vi "WPI_CAN_PDPReceive.vi"(11 "Power Distribution Panel (0)":u8) -> (3 "Power Distribution Panel Out":u8)   [LabVIEW 2017]
uses:
  <vilib>/Rock Robotics/WPI/CAN/PDP/WPI_CAN_PDPMessageIDs.ctl
  <vilib>/Rock Robotics/WPI/CAN/PDP/WPI_CAN_PDPGetAll.ctl
  <vilib>/Rock Robotics/WPI/CAN/PDP/WPI_CAN_PDPGlobalOps.ctl
panel:
  out "Tmeas (ms)":u8
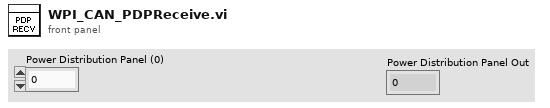
[diagram p1: front panel]
types:
  T1 = typedef "WPI_CAN_PDPMessageIDs.ctl" = u32
  T2 = typedef "WPI_CAN_PDPGetAll.ctl" = cluster{"Channel Currents":dbl[], "Battery Voltage":dbl, "Temperature (degrees C)":dbl, "Internal Battery R (Ohms)":dbl, "Energy (J)":dbl, "Power (W)":dbl, "Total Current (A)":dbl, "CAN Error":errorcluster, "Current Faults":bool[], "Battery Voltage Fault":bool, "Temperature Fault":bool, "Hardware Fault":bool}
  T3 = typedef "WPI_CAN_PDPGlobalOps.ctl" = enum16{"Write After Receive 0-5", "Write After Receive 6-11", "Write After Receive 12-15", "Write After Receive Energy", "Get All", "Get Commands", "Write Clear Sticky Faults Command", "Write Reset Energy Command", "Write Tare Currents Command", "Write Error", "Write After Receive Faults"}
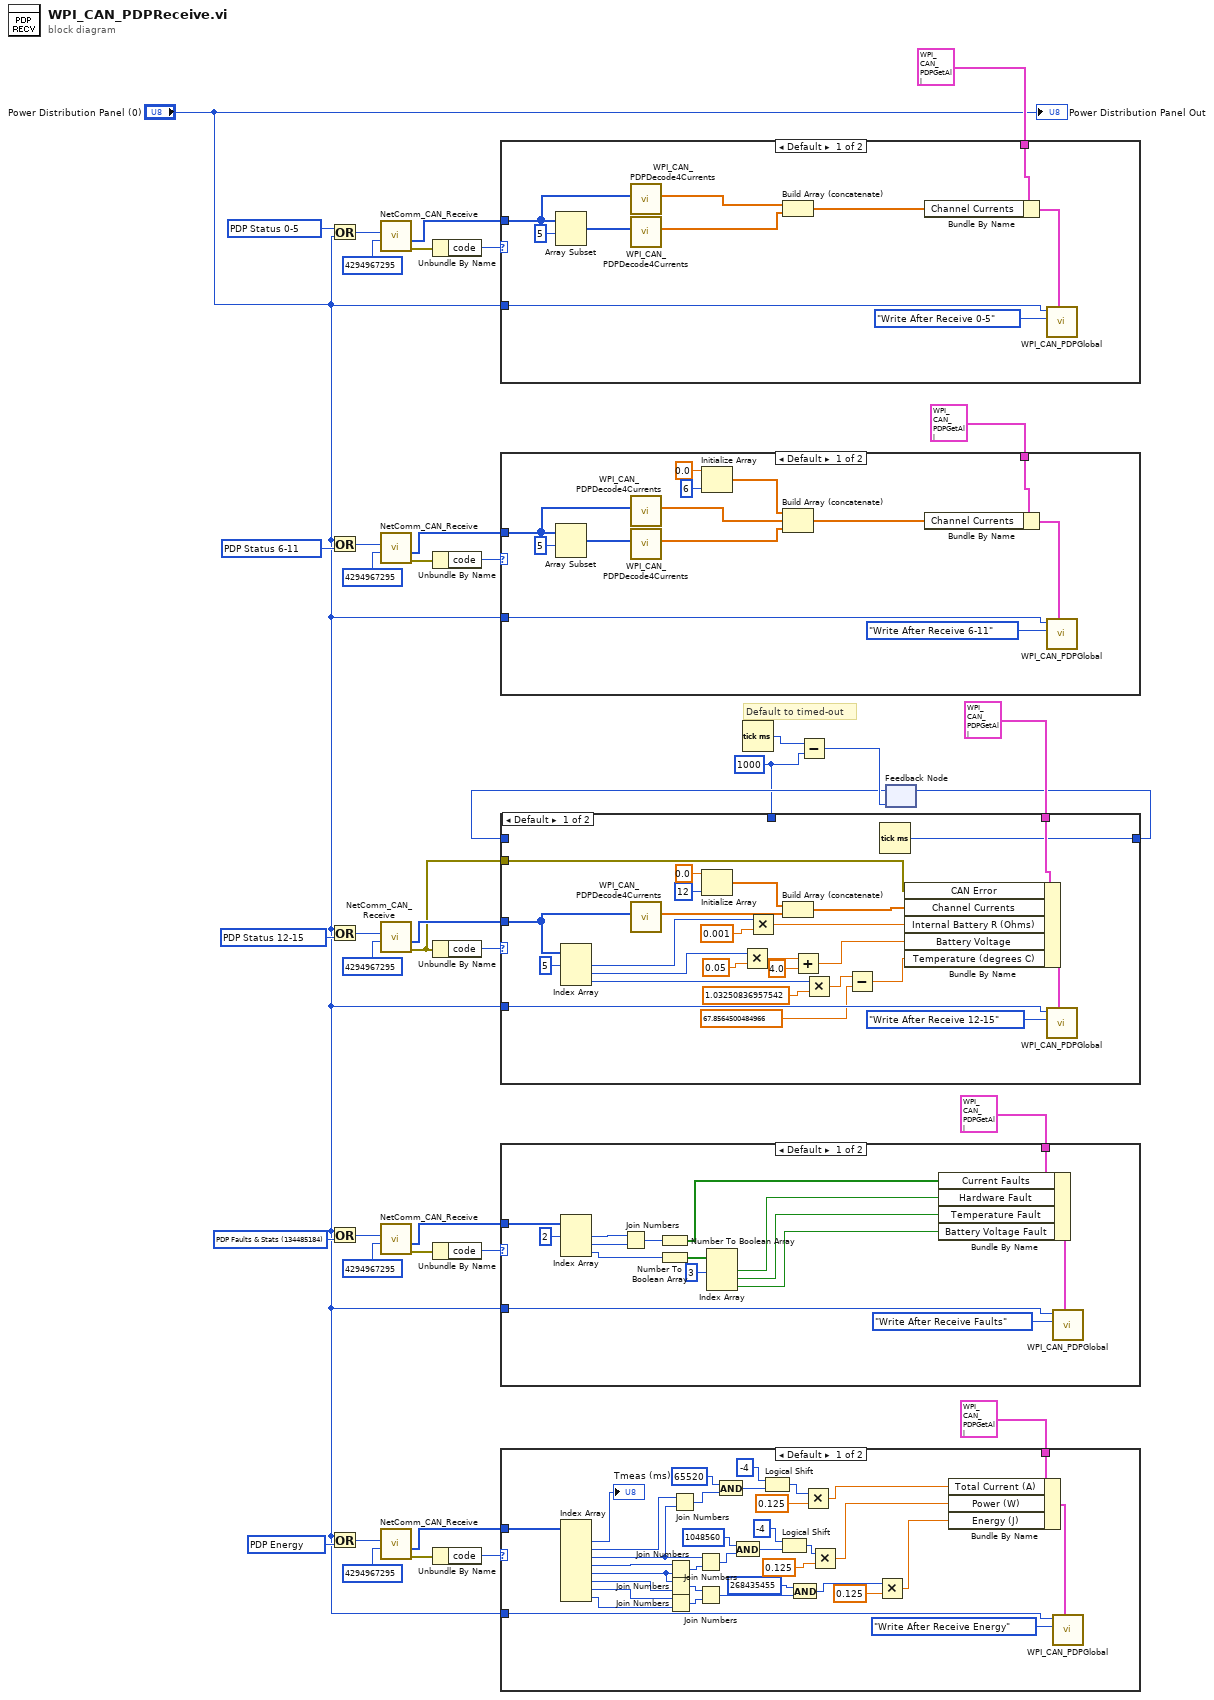
[diagram p0: block diagram]
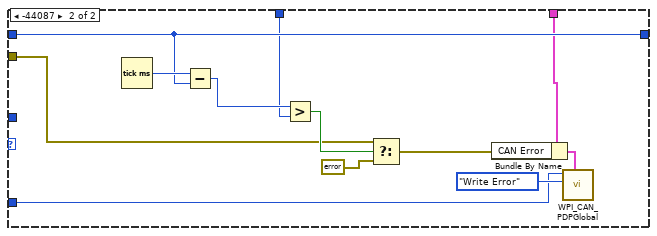
[diagram p4: hidden frame]
diagram:
  w2 = T1 134485184 items=["PDP Status 0-5"=134484992, "PDP Status 6-11"=134485056, "PDP Status 12-15"=134485120, "PDP Faults & Stats"=134485184, "PDP Energy"=134485824, "PDP Commands"=134487040, "PDP Update Event"=134487168, "PDP Update Robot State"=134487104] ("PDP Message IDs")
  w9 = u32 1000 ("y")
  w20 = T1 134485824 items=["PDP Status 0-5"=134484992, "PDP Status 6-11"=134485056, "PDP Status 12-15"=134485120, "PDP Faults & Stats"=134485184, "PDP Energy"=134485824, "PDP Commands"=134487040, "PDP Update Event"=134487168, "PDP Update Robot State"=134487104] ("PDP Message IDs")
  w21 = T1 134485120 items=["PDP Status 0-5"=134484992, "PDP Status 6-11"=134485056, "PDP Status 12-15"=134485120, "PDP Faults & Stats"=134485184, "PDP Energy"=134485824, "PDP Commands"=134487040, "PDP Update Event"=134487168, "PDP Update Robot State"=134487104] ("PDP Message IDs")
  w22 = T1 134485056 items=["PDP Status 0-5"=134484992, "PDP Status 6-11"=134485056, "PDP Status 12-15"=134485120, "PDP Faults & Stats"=134485184, "PDP Energy"=134485824, "PDP Commands"=134487040, "PDP Update Event"=134487168, "PDP Update Robot State"=134487104] ("PDP Message IDs")
  w23 = T1 134484992 items=["PDP Status 0-5"=134484992, "PDP Status 6-11"=134485056, "PDP Status 12-15"=134485120, "PDP Faults & Stats"=134485184, "PDP Energy"=134485824, "PDP Commands"=134487040, "PDP Update Event"=134487168, "PDP Update Robot State"=134487104] ("PDP Message IDs")
  # "Default to timed-out"
  n1 = Or(x=w23, y="Power Distribution Panel (0)") -> (x .or. y?=w41:T1)
  n2 = Or(x="Power Distribution Panel (0)", y=w22) -> (x .or. y?=w25:T1)
  n3 = Or(x="Power Distribution Panel (0)", y=w21) -> (x .or. y?=w24:T1)
  n4 = Or(x="Power Distribution Panel (0)", y=w2) -> (x .or. y?=w3:T1)
  n5 = Or(x="Power Distribution Panel (0)", y=w20) -> (x .or. y?=w19:T1)
  n6 = call <vilib>:"NetComm_CAN_Receive.vi"("Message ID Mask"=u32 4294967295, "Message ID"=w41) -> ("error out"=w39:errorcluster, "Data"=w33:u8[])  [unwired: 6 in, 2 out]
  n7 = call <vilib>:"NetComm_CAN_Receive.vi"("Message ID Mask"=u32 4294967295, "Message ID"=w25) -> ("error out"=w37:errorcluster, "Data"=w35:u8[])  [unwired: 6 in, 2 out]
  n8 = call <vilib>:"NetComm_CAN_Receive.vi"("Message ID Mask"=u32 4294967295, "Message ID"=w24) -> ("error out"=w26:errorcluster, "Data"=w31:u8[])  [unwired: 6 in, 2 out]
  n9 = call <vilib>:"NetComm_CAN_Receive.vi"("Message ID Mask"=u32 4294967295, "Message ID"=w3) -> ("error out"=w4:errorcluster, "Data"=w8:u8[])  [unwired: 6 in, 2 out]
  n10 = call <vilib>:"NetComm_CAN_Receive.vi"("Message ID Mask"=u32 4294967295, "Message ID"=w19) -> ("error out"=w18:errorcluster, "Data"=w14:u8[])  [unwired: 6 in, 2 out]
  n11 = Unbundle By Name(w39) -> ("code"=w34:i32)
  n12 = Unbundle By Name(w37) -> ("code"=w36:i32)
  n13 = Unbundle By Name(w26) -> ("code"=w30:i32)
  n14 = Unbundle By Name(w4) -> ("code"=w7:i32)
  n15 = Unbundle By Name(w18) -> ("code"=w15:i32)
  n16 = case shown="Default" w34 {
    tunnel: "Power Distribution Panel (0)" -> [w50 _]
    tunnel: w33 -> [w43 _]
    tunnel: T2 {"Channel Currents"=[], "Battery Voltage"=0.0, "Temperature (degrees C)"=0.0, "Internal Battery R (Ohms)"=0.0, "Energy (J)"=0.0, "Power (W)"=0.0, "Total Current (A)"=0.0, "CAN Error"={"status"=FALSE, "code"=0, "source"=""}, "Current Faults"=[], "Battery Voltage Fault"=FALSE, "Temperature Fault"=FALSE, "Hardware Fault"=FALSE} ("Write After Receive") -> [w42 _]
    frame Default {
      n17 = Array Subset(array=w43, index=5) -> (w47:u8[])  [unwired: 1 in]
      n18 = call <vilib>:"WPI_CAN_PDPDecode4Currents.vi"("5-Byte Array"=w43) -> ("4-Current Array"=w45:dbl[])  [unwired: 10 in]
      n19 = call <vilib>:"WPI_CAN_PDPDecode4Currents.vi"("5-Byte Array"=w47) -> ("4-Current Array"=w46:dbl[])  [unwired: 10 in]
      n20 = Build Array (concatenate)(w45, w46) -> (w44:dbl[])
      n21 = Bundle By Name(cluster=w42, "Channel Currents"=w44) -> (w49:T2)
      n22 = call <vilib>:"WPI_CAN_PDPGlobal.vi"("Write After Receive"=w49, "Operation"=WPI_CAN_PDPGlobalOps."Write After Receive 0-5", "Power Distribution Panel (0)"=w50) -> ()  [unwired: 6 in, 3 out]
    }
    frame -44087 {
    }
  }
  n23 = case shown="Default" w36 {
    tunnel: w35 -> [w59 _]
    tunnel: "Power Distribution Panel (0)" -> [w63 _]
    tunnel: T2 {"Channel Currents"=[], "Battery Voltage"=0.0, "Temperature (degrees C)"=0.0, "Internal Battery R (Ohms)"=0.0, "Energy (J)"=0.0, "Power (W)"=0.0, "Total Current (A)"=0.0, "CAN Error"={"status"=FALSE, "code"=0, "source"=""}, "Current Faults"=[], "Battery Voltage Fault"=FALSE, "Temperature Fault"=FALSE, "Hardware Fault"=FALSE} ("Write After Receive") -> [w62 _]
    frame Default {
      n24 = Array Subset(array=w59, index=5) -> (w58:u8[])  [unwired: 1 in]
      n25 = call <vilib>:"WPI_CAN_PDPDecode4Currents.vi"("5-Byte Array"=w59) -> ("4-Current Array"=w54:dbl[])  [unwired: 10 in]
      n26 = call <vilib>:"WPI_CAN_PDPDecode4Currents.vi"("5-Byte Array"=w58) -> ("4-Current Array"=w56:dbl[])  [unwired: 10 in]
      n27 = Initialize Array(0.0 ("element"), 6 ("dimension size")) -> (w55:dbl[])
      n28 = Build Array (concatenate)(w55, w54, w56) -> (w52:dbl[])
      n29 = Bundle By Name(cluster=w62, "Channel Currents"=w52) -> (w61:T2)
      n30 = call <vilib>:"WPI_CAN_PDPGlobal.vi"("Write After Receive"=w61, "Operation"=WPI_CAN_PDPGlobalOps."Write After Receive 6-11", "Power Distribution Panel (0)"=w63) -> ()  [unwired: 6 in, 3 out]
    }
    frame -44087 {
    }
  }
  n31 = case shown="Default" w7 {
    tunnel: w8 -> [w76 _]
    tunnel: "Power Distribution Panel (0)" -> [w79 _]
    tunnel: T2 {"Channel Currents"=[], "Battery Voltage"=0.0, "Temperature (degrees C)"=0.0, "Internal Battery R (Ohms)"=0.0, "Energy (J)"=0.0, "Power (W)"=0.0, "Total Current (A)"=0.0, "CAN Error"={"status"=FALSE, "code"=0, "source"=""}, "Current Faults"=[], "Battery Voltage Fault"=FALSE, "Temperature Fault"=FALSE, "Hardware Fault"=FALSE} ("Write After Receive") -> [w78 _]
    frame Default {
      n32 = Index Array(array=w76, index #1=2 ("index")) -> (element #1=w75:u8, element #2=w74:u8, element #3=w70:u8)  [unwired: 2 in]
      n33 = Join Numbers(hi=w75, lo=w74) -> ((hi.lo)=w73:u16)
      n34 = Number To Boolean Array(number=w73) -> (Boolean array=w72:bool[])
      n35 = Number To Boolean Array(number=w70) -> (Boolean array=w69:bool[])
      n36 = Index Array(array=w69, index #1=3 ("index")) -> (element #1=w67:bool, element #2=w66:bool, element #3=w65:bool)  [unwired: 2 in]
      n37 = Bundle By Name(cluster=w78, "Current Faults"=w72, "Hardware Fault"=w67, "Temperature Fault"=w66, "Battery Voltage Fault"=w65) -> (w77:T2)
      n38 = call <vilib>:"WPI_CAN_PDPGlobal.vi"("Write After Receive"=w77, "Operation"=WPI_CAN_PDPGlobalOps."Write After Receive Faults", "Power Distribution Panel (0)"=w79) -> ()  [unwired: 6 in, 3 out]
    }
    frame -44087 {
    }
  }
  n39 = case shown="Default" w15 {
    tunnel: w14 -> [w111 _]
    tunnel: "Power Distribution Panel (0)" -> [w114 _]
    tunnel: T2 {"Channel Currents"=[], "Battery Voltage"=0.0, "Temperature (degrees C)"=0.0, "Internal Battery R (Ohms)"=0.0, "Energy (J)"=0.0, "Power (W)"=0.0, "Total Current (A)"=0.0, "CAN Error"={"status"=FALSE, "code"=0, "source"=""}, "Current Faults"=[], "Battery Voltage Fault"=FALSE, "Temperature Fault"=FALSE, "Hardware Fault"=FALSE} ("Write After Receive") -> [w113 _]
    frame Default {
      n40 = Index Array(array=w111) -> (element #1=→"Tmeas (ms)":u8, element #2=w108:u8, element #3=w99:u8, element #4=w100:u8, element #5=w89:u8, element #6=w88:u8, element #7=w90:u8, element #8=w91:u8)  [unwired: 8 in]
      n41 = Join Numbers(hi=w100, lo=w89) -> ((hi.lo)=w98:u16)
      n42 = Join Numbers(hi=w89, lo=w88) -> ((hi.lo)=w86:u16)
      n43 = Join Numbers(hi=w90, lo=w91) -> ((hi.lo)=w87:u16)
      n44 = Join Numbers(hi=w108, lo=w99) -> ((hi.lo)=w107:u16)
      n45 = Join Numbers(hi=w99, lo=w98) -> ((hi.lo)=w94:u32)
      n46 = Join Numbers(hi=w86, lo=w87) -> ((hi.lo)=w84:u32)
      n47 = And(x=u16 65520, y=w107) -> (x .and. y?=w103:u16)
      n48 = And(x=u32 1048560, y=w94) -> (x .and. y?=w96:u32)
      n49 = Logical Shift(y=i16 -4, x=w103) -> (x << y=w102:u16)
      n50 = Logical Shift(y=i16 -4, x=w96) -> (x << y=w93:u32)
      n51 = And(x=u32 268435455, y=w84) -> (x .and. y?=w82:u32)
      n52 = Multiply(x=w102, y=0.125 ("element")) -> (x*y=w104:dbl)
      n53 = Multiply(x=w93, y=0.125 ("element")) -> (x*y=w92:dbl)
      n54 = Multiply(x=w82, y=0.125 ("element")) -> (x*y=w81:dbl)
      n55 = Bundle By Name(cluster=w113, "Total Current (A)"=w104, "Power (W)"=w92, "Energy (J)"=w81) -> (w112:T2)
      n56 = call <vilib>:"WPI_CAN_PDPGlobal.vi"("Write After Receive"=w112, "Operation"=WPI_CAN_PDPGlobalOps."Write After Receive Energy", "Power Distribution Panel (0)"=w114) -> ()  [unwired: 6 in, 3 out]
    }
    frame -44087 {
    }
  }
  n57 = Tick Count (ms)() -> (millisecond timer value=w13:u32)
  n58 = Subtract(x=w13, y=w9) -> (x-y=w12:u32)
  n59 = feedback #1(w12) -> (w10:u32)
  n60 = case shown="Default" w30 {
    tunnel: w31 -> [w132 _]
    tunnel: "Power Distribution Panel (0)" -> [w140 w142]
    tunnel: T2 {"Channel Currents"=[], "Battery Voltage"=0.0, "Temperature (degrees C)"=0.0, "Internal Battery R (Ohms)"=0.0, "Energy (J)"=0.0, "Power (W)"=0.0, "Total Current (A)"=0.0, "CAN Error"={"status"=FALSE, "code"=0, "source"=""}, "Current Faults"=[], "Battery Voltage Fault"=FALSE, "Temperature Fault"=FALSE, "Hardware Fault"=FALSE} ("Write After Receive") -> [w139 w145]
    tunnel: w26 -> [w130 w147]
    tunnel: [w116 w149] -> w11
    tunnel: w10 -> [_ w149]
    tunnel: w9 -> [_ w148]
    frame Default {
      n61 = Index Array(array=w132, index #1=5 ("index")) -> (element #1=w125:u8, element #2=w123:u8, element #3=w122:u8)  [unwired: 2 in]
      n62 = call <vilib>:"WPI_CAN_PDPDecode4Currents.vi"("5-Byte Array"=w132) -> ("4-Current Array"=w135:dbl[])  [unwired: 10 in]
      n63 = Initialize Array(0.0 ("element"), 12 ("dimension size")) -> (w136:dbl[])
      n64 = Multiply(x=w123, y=0.05 ("element")) -> (x*y=w121:dbl)
      n65 = Multiply(x=w125, y=0.001 ("element")) -> (x*y=w124:dbl)
      n66 = Build Array (concatenate)(w136, w135) -> (w133:dbl[])
      n67 = Add(x=w121, y=4.0 ("x")) -> (x+y=w118:dbl)
      n68 = Multiply(x=w122, y=1.03250836957542 ("element")) -> (x*y=w129:dbl)
      n69 = Subtract(x=w129, y=67.8564500484966 ("x")) -> (x-y=w120:dbl)
      n70 = Tick Count (ms)() -> (millisecond timer value=w116:u32)
      n71 = Bundle By Name(cluster=w139, "CAN Error"=w130, "Channel Currents"=w133, "Internal Battery R (Ohms)"=w124, "Battery Voltage"=w118, "Temperature (degrees C)"=w120) -> (w138:T2)
      n72 = call <vilib>:"WPI_CAN_PDPGlobal.vi"("Write After Receive"=w138, "Operation"=WPI_CAN_PDPGlobalOps."Write After Receive 12-15", "Power Distribution Panel (0)"=w140) -> ()  [unwired: 6 in, 3 out]
    }
    frame -44087 {
      n73 = Tick Count (ms)() -> (millisecond timer value=w153:u32)
      n74 = Subtract(x=w153, y=w149) -> (x-y=w152:u32)
      n75 = Greater?(x=w152, y=w148) -> (0:w151:bool)
      n76 = Select(t=w147, s=w151, f=errorcluster {"status"=FALSE, "code"=0, "source"=""}) -> (s? t:f=w143:errorcluster)
      n77 = Bundle By Name(cluster=w145, "CAN Error"=w143) -> (w144:T2)
      n78 = call <vilib>:"WPI_CAN_PDPGlobal.vi"("Write After Receive"=w144, "Operation"=WPI_CAN_PDPGlobalOps."Write Error", "Power Distribution Panel (0)"=w142) -> ()  [unwired: 6 in, 3 out]
    }
  }
  n79 = feedback-in #1(w11) -> ()
  "Power Distribution Panel Out" <- "Power Distribution Panel (0)"
